vi "WPI_SimpleGyro_Loop.vi"(8 "error in":errorcluster, 11 "SimpleGyroDevRef":T1) -> (0 "error out":errorcluster)   [LabVIEW 2014, in "SimpleGyro.lvlib"]
doc: "Periodically reads the SimpleGyro and makes data available to your robot project. Place this block within PeriodicTasks.vi."
uses:
  SimpleGyro.lvlib
  WPI_SimpleGyroDevRef.ctl
  <vilib>/Rock Robotics/SystemInterfaces/Typedef/FPGA_TypedefDigitalModule.ctl
  <vilib>/Rock Robotics/SystemInterfaces/spilib/spi_bus.ctl
  <vilib>/Rock Robotics/WPI/SPI/WPI_SPIDevRef.ctl
  <vilib>/Platform/TimedLoop/XDataNode/timing_clust.ctl
  <vilib>/Platform/TimedLoop/XDataNode/nitl_modes.ctl
  <vilib>/Platform/TimedLoop/XDataNode/wakeup.ctl
  <vilib>/platform/TimedLoop/XDataNode/XDataNode.xnode
  <vilib>/Platform/TimedLoop/XDataNode/XDNodeRunTimeDep.lvlib
  <vilib>/ptbypt/NI_PtbyPt.lvlib
panel:
  out "Rate":dbl
  out "Device Found":bool
  out "Offset":dbl
  out "mean 2":dbl format="%0.2f"
  out "Angle":dbl
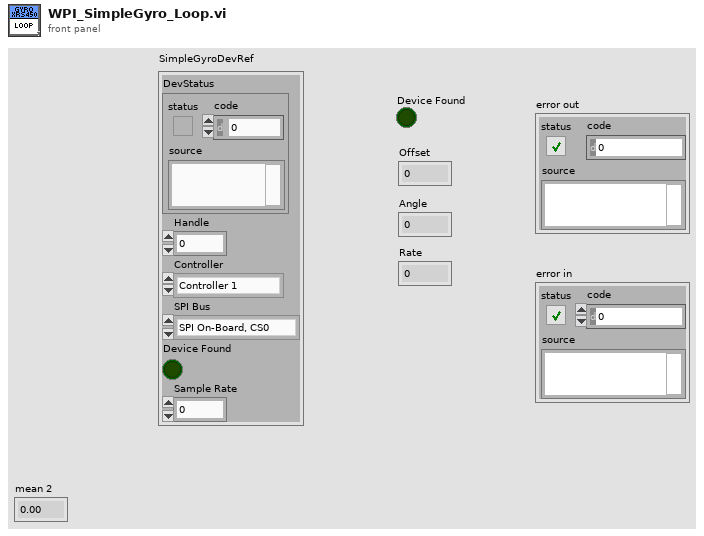
[diagram p1: front panel]
types:
  T1 = typedef "SimpleGyro.lvlib/WPI_SimpleGyroDevRef.ctl" = cluster{"DevStatus":errorcluster, "Handle":i32, "Controller":T2, "SPI Bus":T3, "Device Found":bool, "Sample Rate":dbl}
  T2 = typedef "FPGA_TypedefDigitalModule.ctl" = enum16{"Controller 1"}
  T3 = typedef "spi_bus.ctl" = enum16{"SPI On-Board, CS0", "SPI On-Board, CS1", "SPI On-Board, CS2", "SPI On-Board, CS3", "SPI MXP", "Invalid"}
  T4 = typedef "WPI_SPIDevRef.ctl" = cluster{"DevStatus":errorcluster, "Handle":i32, "Controller":T2, "SPI Bus":T3}
  T5 = typedef "XDNodeRunTimeDep.lvlib/timing_clust.ctl" = cluster{"Expected End [f-1]":u64, "Actual End [f-1]":u64, "Finished Late? [f-1]":bool, "Expected End [i-1]":u64, "Actual End [i-1]":u64, "Finished Late? [i-1]":bool, "Expected Start [i]":u64, "Actual Start [i]":u64, "Expected Start [f]":u64, "Actual Start [f]":u64, "Source Name":string, "Structure Name":string, "Period":i64, "Deadline":i64, "Offset":i64, "Start":i64, "Priority":i32, "Timeout":i32, "Mode":T6, "Wakeup Reason":T7, "Error":errorcluster, "Source Type":string, "Secondary Source Type":string, "Global End Time":u64, "Global Start Time":u64, "Frame Duration":u64, "Iteration Duration":u64, "Assigned CPU":i32, "I/O Scan Engine Mode":u32}
  T6 = typedef "XDNodeRunTimeDep.lvlib/nitl_modes.ctl" = enum32{"No Change", "Process missed periods, maintain original phase", "Discard missed periods, maintain original phase", "Process missed periods, ignore original phase", "Discard missed periods, ignore original phase"}
  T7 = typedef "XDNodeRunTimeDep.lvlib/wakeup.ctl" = enum32{"Normal", "Aborted", "Asynchronous wakeup", "Timing source error", "Timed loop error", "Timeout"}
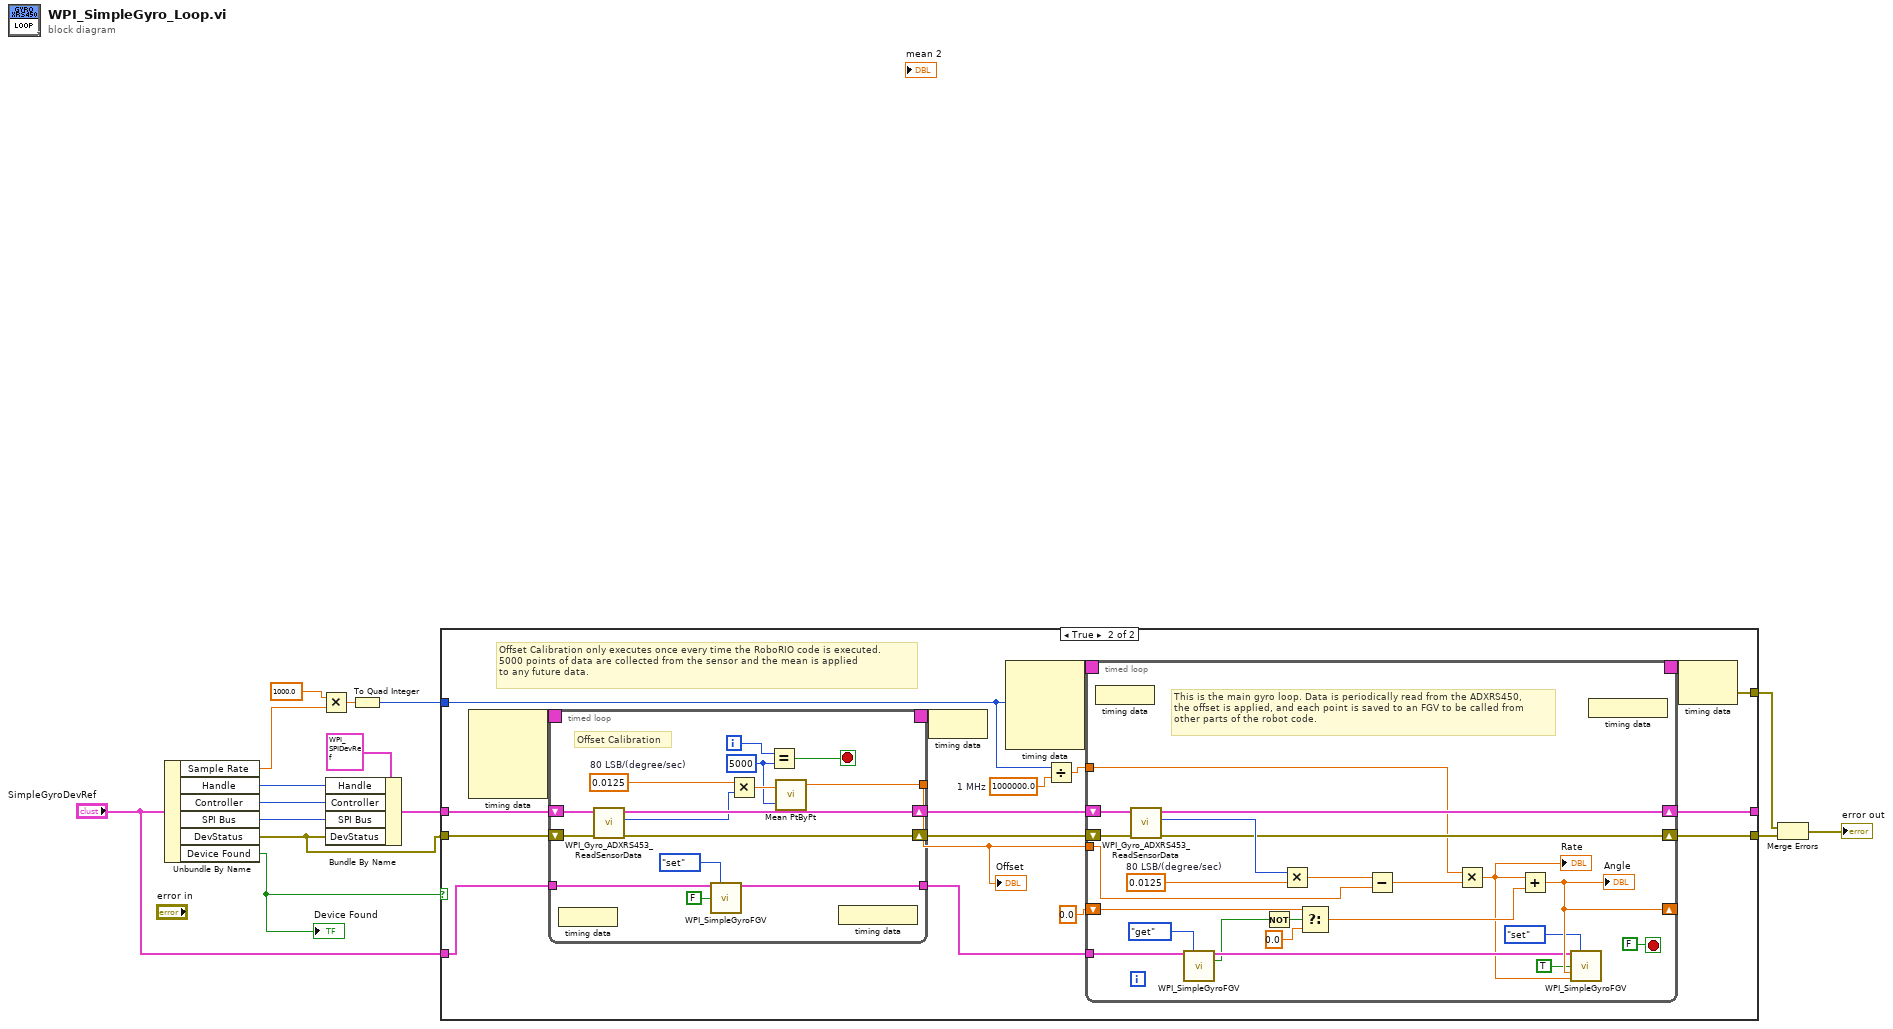
[diagram p0: block diagram]
diagram:
  n1 = Unbundle By Name("SimpleGyroDevRef") -> ("Sample Rate"=w4:dbl, "Handle"=w14:i32, "Controller"=w13:T2, "SPI Bus"=w12:T3, "DevStatus"=w1:errorcluster, "Device Found"=w11:bool)
  "Device Found" <- w11
  n2 = Multiply(x=1000.0 ("y"), y=w4) -> (x*y=w10:dbl)
  n3 = Bundle By Name(cluster=T4 {"DevStatus"={"status"=FALSE, "code"=0, "source"=""}, "Handle"=0, "Controller"=enum."Controller 1", "SPI Bus"=enum."Invalid"} ("SPIDevRef out"), "Handle"=w14, "Controller"=w13, "SPI Bus"=w12, "DevStatus"=w1) -> (w2:T4)
  n4 = To Quad Integer(1:w10) -> (0:w9:i64)
  n5 = case shown="True" w11 {
    tunnel: w2 -> [w17 w24]
    tunnel: w1 -> [w16 w23]
    tunnel: [w16 w33] -> w7
    tunnel: [w17 w32] -> _
    tunnel: w9 -> [_ w30]
    tunnel: "SimpleGyroDevRef" -> [_ w19]
    tunnel: [_ w29] -> w6
    frame False {
    }
    frame True {
      w27 = 1000000.0  # 1 MHz
      # "Offset Calibration only executes once every time the RoboRIO code is executed.\n5000 points of data are collected from the sensor and the mean is applied\nto any future data."
      n6 = node-c288() -> (w26:T5)  [unwired: 4 in]
      n7 = timed-loop {
        shift-right: [w48] -> w22
        shift-left: w24 -> [w50]
        shift-right: [w45] -> w21
        shift-left: w23 -> [w49]
        timing: w26 -> [_]
        timing-out: [_] -> w25
        tunnel: [w43] -> w20
        tunnel: w19 -> [w38]
        tunnel: [w36] -> w18
        i -> [w42]
        stop <- w40 stop-if-true
        w41 = 5000 ("y")
        w46 = 0.0125  # 80 LSB/(degree/sec)
        # "Offset Calibration"
        n8 = node-c288() -> ()  [unwired: 1 in]
        n9 = call "WPI_Gyro_ADXRS453_ReadSensorData.vi"("error in (no error)"=w49, "SPIDevRef in"=w50) -> ("error out"=w45:errorcluster, "Sensor Data (n-1)"=w47:i16, "SPIDevRef out"=w48:T4)  [unwired: 5 in, 2 out]
        n10 = call "WPI_SimpleGyroFGV.vi"("SimpleGyroDevRef"=w38, "Operation"=enum16{"set", "get"}."set", "Calibrated"=FALSE) -> ("SimpleGyroDevRef"=w36:T1)  [unwired: 8 in, 4 out]
        n11 = Multiply(x=w46, y=w47) -> (x*y=w44:dbl)
        n12 = Equal?(x=w42, y=w41) -> (x = y?=w40:bool)
        n13 = call <vilib>:"Mean PtByPt.vi"("x"=w44, "sample length"=w41) -> ("mean"=w43:dbl)  [unwired: 2 in, 1 out]
        n14 = node-c288() -> ()  [unwired: 1 out]
      }
      "Offset" <- w20
      n15 = node-c288(w25) -> ()
      n16 = node-c288(w30) -> (w35:T5)  [unwired: 3 in]
      n17 = Divide(x=w30, y=w27) -> (x/y=w31:dbl)
      n18 = timed-loop {
        shift-right: [w75] -> w32
        shift-left: w22 -> [w77]
        shift-right: [w71] -> w33
        shift-left: w21 -> [w76]
        timing: w35 -> [_]
        timing-out: [_] -> w34
        shift-right: [w64] -> _
        shift-left: 0.0 -> [w72]
        tunnel: w31 -> [w60]
        tunnel: w18 -> [w66]
        tunnel: w20 -> [w58]
        stop <- FALSE stop-if-true
        w73 = 0.0125  # 80 LSB/(degree/sec)
        # "This is the main gyro loop. Data is periodically read from the ADXRS450, \nthe offset is applied, and each point is saved to an FGV to be called from\nother parts of the robot code."
        n19 = node-c288() -> ()  [unwired: 1 in]
        n20 = call "WPI_Gyro_ADXRS453_ReadSensorData.vi"("error in (no error)"=w76, "SPIDevRef in"=w77) -> ("error out"=w71:errorcluster, "Sensor Data (n-1)"=w74:i16, "SPIDevRef out"=w75:T4)  [unwired: 5 in, 2 out]
        n21 = call "WPI_SimpleGyroFGV.vi"("SimpleGyroDevRef"=w66, "Operation"=enum16{"set", "get"}."get") -> ("SimpleGyroDevRef"=w62:T1, "Reset?"=w61:bool)  [unwired: 9 in, 3 out]
        n22 = Not(x=w61) -> (.not. x?=w67:bool)
        n23 = Multiply(x=w74, y=w73) -> (x*y=w59:dbl)
        n24 = Select(t=w72, s=w67, f=0.0 ("t")) -> (s? t:f=w69:dbl)
        n25 = Subtract(x=w59, y=w58) -> (x-y=w57:dbl)
        n26 = Multiply(x=w60, y=w57) -> (x*y=w56:dbl)
        "Rate" <- w56
        n27 = Add(x=w56, y=w69) -> (x+y=w64:dbl)
        "Angle" <- w64
        n28 = call "WPI_SimpleGyroFGV.vi"("SimpleGyroDevRef"=w62, "Operation"=enum16{"set", "get"}."set", "Calibrated"=TRUE, "Angle"=w64, "Rate"=w56) -> ()  [unwired: 6 in, 5 out]
        n29 = node-c288() -> ()  [unwired: 1 out]
      }
      n30 = node-c288(w34) -> (w29:errorcluster)
    }
  }
  n31 = Merge Errors(w6, w7) -> (→"error out":errorcluster)
